vi "Parse Bus Monitor.vi"(8 "error in (no error)":errorcluster, 11 "Bus Monitor XML Node":refnum<k20>) -> (0 "error out":errorcluster, 3 "Bus Monitor":refnum<class "Bus Monitor.lvclass">[](array[class]))   [LabVIEW 2016]
doc: "Retireves all the Filters from the Bus Monitor XML node. Additionally provides a default configuration for other Bus Monitor parameters."
uses:
  Bus Monitor/Bus Monitor.lvclass
  Bus Monitor/TypeDefs/Bus Monitor Configuration.ctl
  <vilib>/xml/NI_XML.lvlib
  Filters/Filter/Filter.lvclass
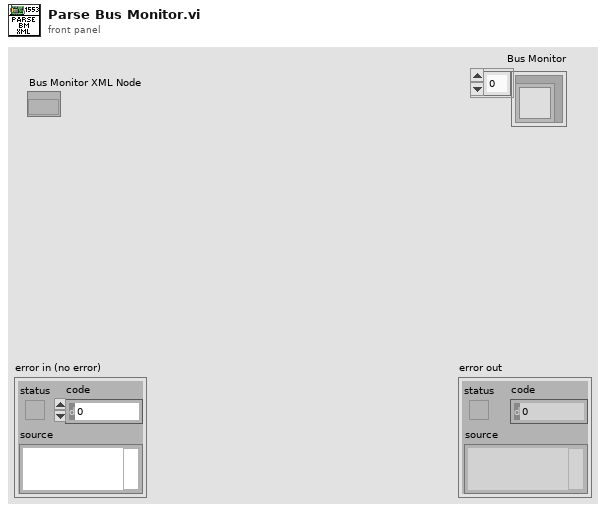
[diagram p1: front panel]
types:
  T1 = typedef "BCI-1553 API.lvlib/Bus Monitor.lvclass/Bus Monitor Configuration.ctl" = cluster{"BM Timeout":u8, "Gap Check":bool, "BM Time Tag Msg Bit Select":u8, "BM Start Record Req":u8, "Cont Record After Inv Word":bool, "Ext Msg Flag Enable":bool, "48-bit Time Tag":bool}
  T2 = typedef "BCI-1553 API.lvlib/1553 SubComponent.lvclass/Parameter Table Data.ctl" = cluster{"Parameter Name":string, "Base Word":u16, "Address":u16, "Value":u64, "Mask":u16[], "Scaling Info":T3}
  T3 = typedef "BCI-1553 API.lvlib/1553 SubComponent.lvclass/Scaling Information.ctl" = cluster{"Bit Offset":i32, "Bit Count":i32, "LSB Resolution":dbl, "2's Complement":bool, "Big Endian":bool, "Sign Bit":bool}
  T4 = typedef "BCI-1553 API.lvlib/Filter Configuration.ctl" = cluster{"Filter Type":T5, "Terminal Address (0-30)":u16, "SubAddress (1-30)":u16, "Mode Code":bool, "Broadcast":bool, "RT-RT":bool, "Bus A":bool}
  T5 = typedef "BCI-1553 API.lvlib/Command Type.ctl" = enum16{"Transmit", "Receive"}
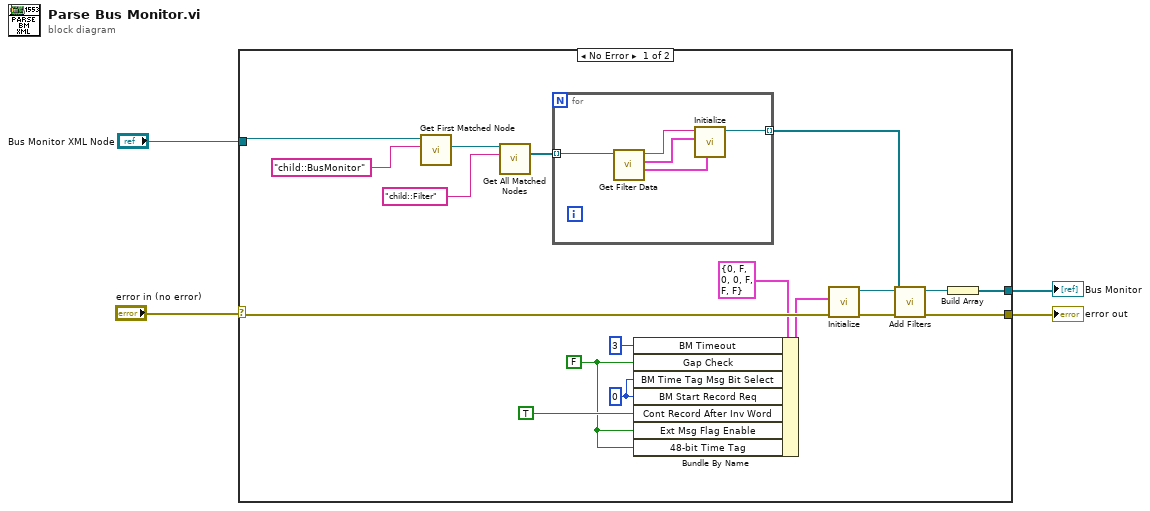
[diagram p0: block diagram]
diagram:
  n1 = case shown="No Error" "error in (no error)" {
    selector: "error in (no error)" -> [w22 w28]
    tunnel: [w12 w28] -> w3
    tunnel: [w21 _] -> w2
    tunnel: "Bus Monitor XML Node" -> [w20 _]
    frame No Error {
      w7 = u8 0 ("BM Start Record Req")
      w5 = FALSE ("Gap Check")
      n2 = call <vilib>:"Get First Matched Node.vi"("XPath expression"="child::BusMonitor", "node in"=w20) -> ("node result"=w19:refnum<k20>)  [unwired: 7 in, 2 out]
      n3 = call <vilib>:"Get All Matched Nodes.vi"("XPath expression"="child::Filter", "node in"=w19) -> ("node result array"=w18:refnum<k20>[])  [unwired: 7 in, 2 out]
      n4 = for {
        tunnel: w18 -> [w26] mode=indexing
        tunnel: [w27] -> w15 mode=indexing
        n5 = call "Get Filter Data.vi"("Filter XML Ref"=w26) -> ("Parameters"=w23:T2[], "Filter Configuration"=w24:T4, "Name"=w25:string)  [unwired: 7 in, 1 out]
        n6 = call "Initialize.vi"("Parameters"=w23, "Filter Configuration"=w24, "ID"=w25) -> ("Filter out"=w27:refnum<class "Filter.lvclass">)  [unwired: 7 in, 1 out]
      }
      n7 = Bundle By Name(cluster=T1 {"BM Timeout"=0, "Gap Check"=FALSE, "BM Time Tag Msg Bit Select"=0, "BM Start Record Req"=0, "Cont Record After Inv Word"=FALSE, "Ext Msg Flag Enable"=FALSE, "48-bit Time Tag"=FALSE} ("Bus Monitor Configuration"), "BM Timeout"=u8 3, "Gap Check"=w5, "BM Time Tag Msg Bit Select"=w7, "BM Start Record Req"=w7, "Cont Record After Inv Word"=TRUE, "Ext Msg Flag Enable"=w5, "48-bit Time Tag"=w5) -> (w9:T1)
      n8 = call "Initialize.vi"("error in (no error)"=w22, "Bus Monitor Configuration"=w9) -> ("error out"=w13:errorcluster, "Bus Monitor out"=w14:refnum<class "Bus Monitor.lvclass">)  [unwired: 8 in]
      n9 = call-dynamic "Add Filters.vi"("error in (no error)"=w13, "Filters"=w15, "Bus Monitor in"=w14) -> ("error out"=w12:errorcluster, "Bus Monitor out"=w11:refnum<class "Bus Monitor.lvclass">)  [unwired: 7 in]
      n10 = Build Array(w11) -> (w21:refnum<class "Bus Monitor.lvclass">[])
    }
    frame Error {
    }
  }
  "error out" <- w3
  "Bus Monitor" <- w2
